vi "Update Map.vi"(9 "Action":T2, 10 "Direction":T1, 11 "Class":refnum<class "Cautious Wolf.lvclass">) -> (3 "Class":refnum<class "Cautious Wolf.lvclass">)   [LabVIEW 2015, in "Cautious Wolf.lvclass"]
uses:
  Cautious Wolf.lvclass
  Type Defs/Action Enum.ctl
  Type Defs/Direction Enum.ctl
  Cautious Wolf.lvclass/Cautious Wolf.ctl
  SubVIs/Read-Only Globals.vi
  Square/Square.lvclass
  Type Defs/SB Type Defs.lvlib
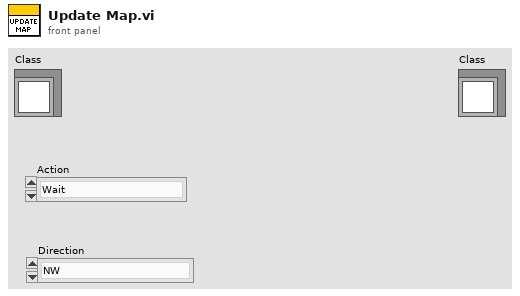
[diagram p1: front panel]
types:
  T1 = typedef "SB Type Defs.lvlib/Direction Enum.ctl" = enum16{"NW", "N", "NE", "E", "SE", "S", "SW", "W"}
  T2 = typedef "SB Type Defs.lvlib/Action Enum.ctl" = enum16{"Wait", "Move", "Attack", "Replicate"}
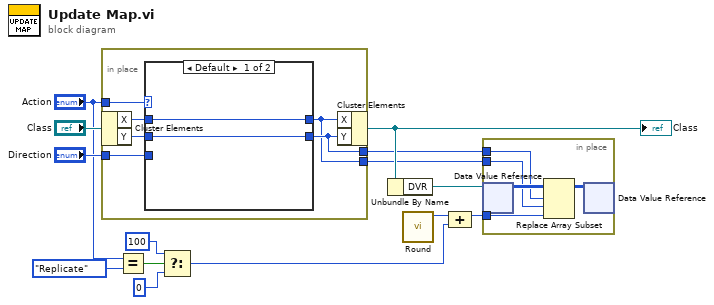
[diagram p0: block diagram]
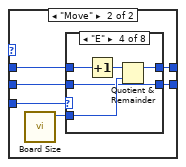
[diagram p2: hidden frame]
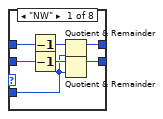
[diagram p3: hidden frame]
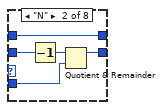
[diagram p4: hidden frame]
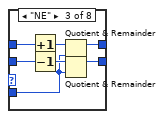
[diagram p5: hidden frame]
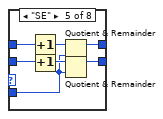
[diagram p6: hidden frame]
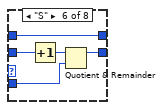
[diagram p7: hidden frame]
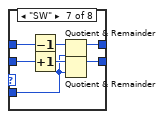
[diagram p8: hidden frame]
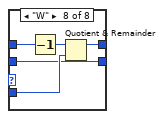
[diagram p9: hidden frame]
diagram:
  n1 = in-place {
    in-place-border: "Direction" -> [w20]
    in-place-border: [w17] -> w10
    in-place-border: [w16] -> w9
    in-place-border: "Action" -> [w15]
    n2 = in-place-cluster #1("Class") -> ("X"=w19:i32, "Y"=w18:i32)
    n3 = case shown="Default" w15 {
      tunnel: w20 -> [_ w28]
      tunnel: w19 -> [w22 w27]
      tunnel: w18 -> [w21 w26]
      tunnel: [w21 w25] -> w17
      tunnel: [w22 w24] -> w16
      frame Default {
      }
      frame "Move" {
        n4 = call "Board Size.vi"() -> ("Board Size"=w23:i32)  [unwired: 11 in]
        n5 = case shown="\"E\"" w28 {
          tunnel: w27 -> [w34 w36 w46 w52 w58 w60 w70 w76]
          tunnel: w26 -> [w35 w40 w47 w48 w59 w64 w71 w72]
          tunnel: [w32 w38 w44 w48 w56 w62 w68 w72] -> w25
          tunnel: [w29 w36 w41 w49 w53 w60 w65 w73] -> w24
          tunnel: w23 -> [w30 w37 w42 w50 w54 w61 w66 w74]
          frame "NW" {
            n6 = Decrement(x=w34) -> (x-1=w31:i32)
            n7 = Decrement(x=w35) -> (x-1=w33:i32)
            n8 = Quotient & Remainder(x=w31, y=w30) -> (x-y*floor(x/y)=w29:i32)  [unwired: 1 out]
            n9 = Quotient & Remainder(x=w33, y=w30) -> (x-y*floor(x/y)=w32:i32)  [unwired: 1 out]
          }
          frame "N" {
            n10 = Decrement(x=w40) -> (x-1=w39:i32)
            n11 = Quotient & Remainder(x=w39, y=w37) -> (x-y*floor(x/y)=w38:i32)  [unwired: 1 out]
          }
          frame "NE" {
            n12 = Increment(x=w46) -> (x+1=w43:i32)
            n13 = Decrement(x=w47) -> (x-1=w45:i32)
            n14 = Quotient & Remainder(x=w43, y=w42) -> (x-y*floor(x/y)=w41:i32)  [unwired: 1 out]
            n15 = Quotient & Remainder(x=w45, y=w42) -> (x-y*floor(x/y)=w44:i32)  [unwired: 1 out]
          }
          frame "E" {
            n16 = Increment(x=w52) -> (x+1=w51:i32)
            n17 = Quotient & Remainder(x=w51, y=w50) -> (x-y*floor(x/y)=w49:i32)  [unwired: 1 out]
          }
          frame "SE" {
            n18 = Increment(x=w58) -> (x+1=w55:i32)
            n19 = Increment(x=w59) -> (x+1=w57:i32)
            n20 = Quotient & Remainder(x=w55, y=w54) -> (x-y*floor(x/y)=w53:i32)  [unwired: 1 out]
            n21 = Quotient & Remainder(x=w57, y=w54) -> (x-y*floor(x/y)=w56:i32)  [unwired: 1 out]
          }
          frame "S" {
            n22 = Increment(x=w64) -> (x+1=w63:i32)
            n23 = Quotient & Remainder(x=w63, y=w61) -> (x-y*floor(x/y)=w62:i32)  [unwired: 1 out]
          }
          frame "SW" {
            n24 = Decrement(x=w70) -> (x-1=w67:i32)
            n25 = Increment(x=w71) -> (x+1=w69:i32)
            n26 = Quotient & Remainder(x=w67, y=w66) -> (x-y*floor(x/y)=w65:i32)  [unwired: 1 out]
            n27 = Quotient & Remainder(x=w69, y=w66) -> (x-y*floor(x/y)=w68:i32)  [unwired: 1 out]
          }
          frame "W" {
            n28 = Decrement(x=w76) -> (x-1=w75:i32)
            n29 = Quotient & Remainder(x=w75, y=w74) -> (x-y*floor(x/y)=w73:i32)  [unwired: 1 out]
          }
        }
      }
    }
    n30 = in-place-cluster #1("X"=w16, "Y"=w17) -> (w13:refnum<class "Cautious Wolf.lvclass">)
  }
  "Class" <- w13
  n31 = Equal?(x="Action", y=Action_Enum."Replicate") -> (x = y?=w5:bool)
  n32 = Select(t=100, s=w5, f=0) -> (s? t:f=w3:i32)
  n33 = Unbundle By Name(w13) -> ("DVR"=w11:refnum<data-value>)
  n34 = call "Round.vi"() -> ("Round"=w8:i32)  [unwired: 11 in]
  n35 = Compound Arithmetic op=ADD(w8, w3) -> (w4:i32)
  n36 = in-place {
    in-place-border: w10 -> [w80]
    in-place-border: w9 -> [w78]
    in-place-border: w4 -> [w77]
    n37 = in-place-dvr #2(w11) -> (w81:i32[][])  [unwired: 1 out]
    n38 = Replace Array Subset(array=w81, new element=w77, index (row)=w80, index (col)=w78) -> (w79:i32[][])
    n39 = in-place-dvr #2(w79) -> ()  [unwired: 2 out]
  }
